vi "Hardware_Power Supplies_Init.vi"(11 "VISA name":refnum<visa-resource-name>="Power_Supplies") -> (0 "Error out":errorcluster, 3 "VISA out":refnum<visa-resource-name>)   [LabVIEW 2017]
panel:
  in  "Error In":errorcluster
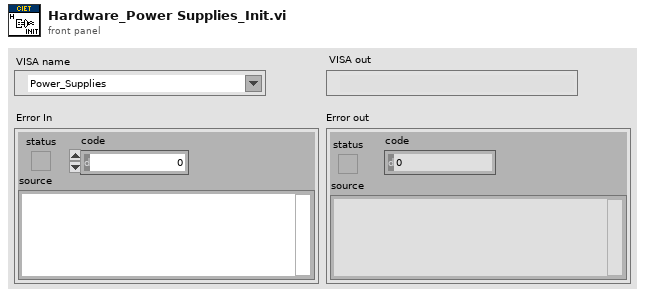
[diagram p1: front panel]
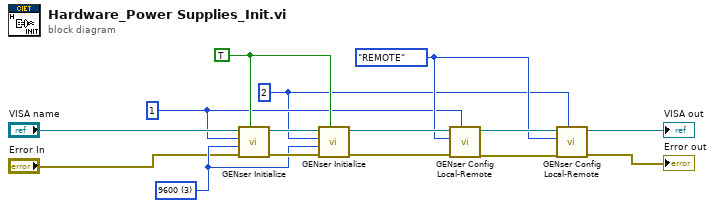
[diagram p0: block diagram]
diagram:
  w4 = enum16{"LOCAL", "REMOTE", "LOCKOUT"}."REMOTE" ("Mode")
  w2 = i16 2 ("GEN Addr")
  w5 = TRUE ("Reset (T)")
  w3 = i16 1 ("GEN Addr")
  w9 = u16 3 items=["1200", "2400", "4800", "9600", "19200"] ("BAUD")
  n1 = call "GENser Initialize.vi"("Reset (T)"=w5, "error in (no error)"="Error In", "BAUD"=w9, "GEN Addr"=w3, "VISA name"="VISA name") -> ("error out"=w14:errorcluster, "VISA out"=w15:refnum<visa-resource-name>)  [unwired: 5 in]
  n2 = call "GENser Initialize.vi"("Reset (T)"=w5, "error in (no error)"=w14, "BAUD"=w9, "GEN Addr"=w2, "VISA name"=w15) -> ("error out"=w12:errorcluster, "VISA out"=w13:refnum<visa-resource-name>)  [unwired: 5 in]
  n3 = call "GENser Config Local-Remote.vi"("GEN Addr"=w3, "error"=w12, "Mode"=w4, "VISA"=w13) -> ("error out"=w10:errorcluster, "VISA out"=w11:refnum<visa-resource-name>)  [unwired: 6 in]
  n4 = call "GENser Config Local-Remote.vi"("GEN Addr"=w2, "error"=w10, "Mode"=w4, "VISA"=w11) -> ("error out"=→"Error out":errorcluster, "VISA out"=→"VISA out":refnum<visa-resource-name>)  [unwired: 6 in]
